vi "_Write_Query.vi"(8 "error in (no error)":errorcluster, 11 "Postgres Connector In":refnum<class "Postgres Connector.lvclass">) -> (0 "error out":errorcluster, 3 "Postgres Connector Out":refnum<class "Postgres Connector.lvclass">)   [LabVIEW 2020, in "Postgres Connector.lvclass"]
doc: "This VI is used to send a command to the PostgreSQL database"
uses:
  Postgres Connector.lvclass
  Postgres Connector.lvclass/Postgres Connector.ctl
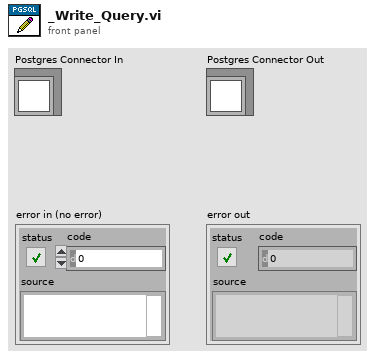
[diagram p1: front panel]
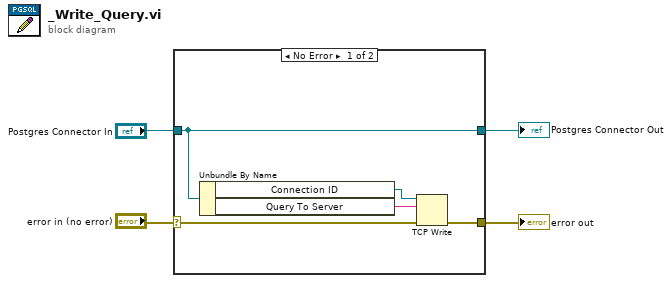
[diagram p0: block diagram]
diagram:
  n1 = case shown="No Error" "error in (no error)" {
    selector: "error in (no error)" -> [w8 w11]
    tunnel: "Postgres Connector In" -> [w5 w10]
    tunnel: [w7 w11] -> w2
    tunnel: [w5 w10] -> w1
    frame No Error {
      n2 = Unbundle By Name(w5) -> ("Connection ID"=w9:refnum<k5>, "Query To Server"=w6:string)
      n3 = TCP Write(connection ID=w9, data in=w6, error in (no error)=w8) -> (error out=w7:errorcluster)  [unwired: 1 in, 2 out]
    }
    frame Error {
    }
  }
  "error out" <- w2
  "Postgres Connector Out" <- w1
